vi "Actor Core.vi"(8 "error in":errorcluster, 11 "State in":refnum<class "System Actor.lvclass">) -> (0 "error out":errorcluster, 3 "Actor out":refnum<class "Actor.lvclass">)   [LabVIEW 2013, in "Robot Actors.lvlib" / "System Actor.lvlib" / "System Actor.lvclass"]
doc: "(<B>Filename</B>: Actor Framework.lvlib:Actor.lvclass:Actor Core.vi)\n\nThis override invokes Entry.vi on the initial state, prior to calling the parent Actor Core. Adding this behavior to Actor Core (instead of an override of Pre Launch Init.vi) allows the initial state to launch a nested actor as part of its entry behavior.\n\nReceives messages to the actor, reacts to them, and initiates any error handling that may shut the actor down.\n\nDescendant classes may override this VI to append parallel tasks for the actor to complete while it handles messages. Overrides use the Call Parent Method node."
uses:
  System Actor.lvclass
  State Actor/State Actor.lvclass
  <vilib>/ActorFramework/Actor/Actor.lvclass
  Command Processor/States/No Command/No Command Class/No Command.lvclass
  System Status.ctl
  Command/Command Class/Command Status.ctl
  Command/Command Class/Command.lvclass
  Command/Command Class/Command States.ctl
  Command Processor/Command Processor Class/Command Processor Status.ctl
  Command Processor/Command Processor Class/Command Processor.lvclass
  Command Processor/Command Processor Class/Command Processor States.ctl
panel:
  out "System Status":T1
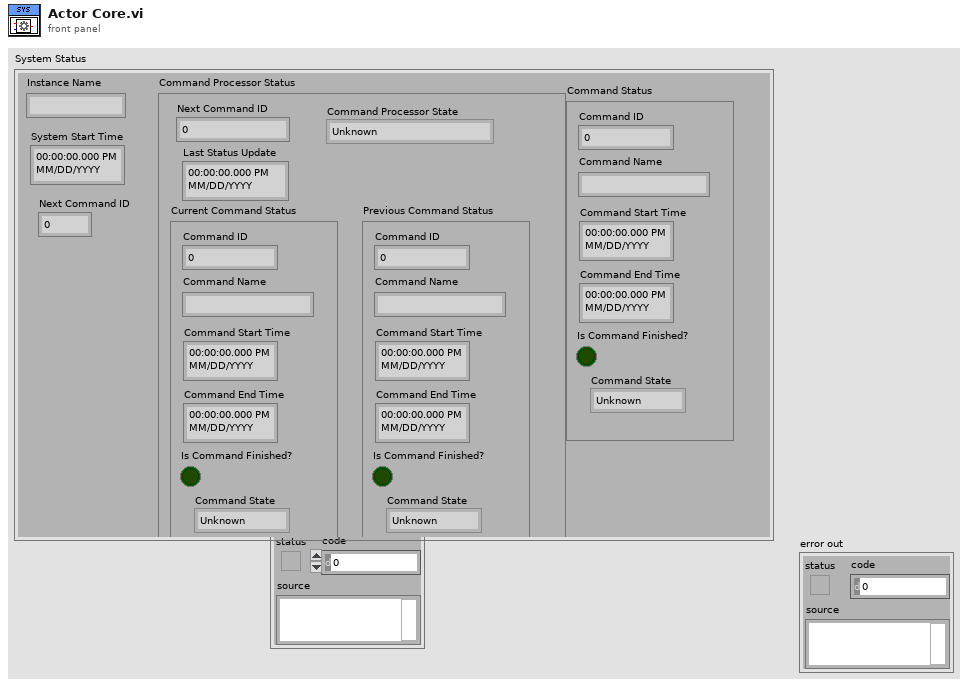
[diagram p1: front panel]
types:
  T1 = typedef "Robot Actors.lvlib/System Actor.lvlib/System Actor.lvclass/System Status.ctl" = cluster{"Instance Name":string, "Command Status":T2, "System Start Time":timestamp, "Next Command ID":dbl, "Command Processor Status":T4}
  T2 = typedef "Robot Actors.lvlib/Command.lvlib/Command.lvclass/Command Status.ctl" = cluster{"Command Name":string, "Command Start Time":timestamp, "Command End Time":timestamp, "Is Command Finished?":bool, "Command ID":dbl, "Command State":T3}
  T3 = typedef "Robot Actors.lvlib/Command.lvlib/Command.lvclass/Command States.ctl" = enum16{"Unknown", "Started", "Stopped", "Finished"}
  T4 = typedef "Robot Actors.lvlib/Command Processor.lvlib/Command Processor.lvclass/Command Processor Status.ctl" = cluster{"Next Command ID":dbl, "Current Command Status":T2, "Previous Command Status ":T2, "Command Processor State":T5, "Last Status Update":timestamp}
  T5 = typedef "Robot Actors.lvlib/Command Processor.lvlib/Command Processor.lvclass/Command Processor States.ctl" = enum16{"Unknown", "No Command", "Running Command"}
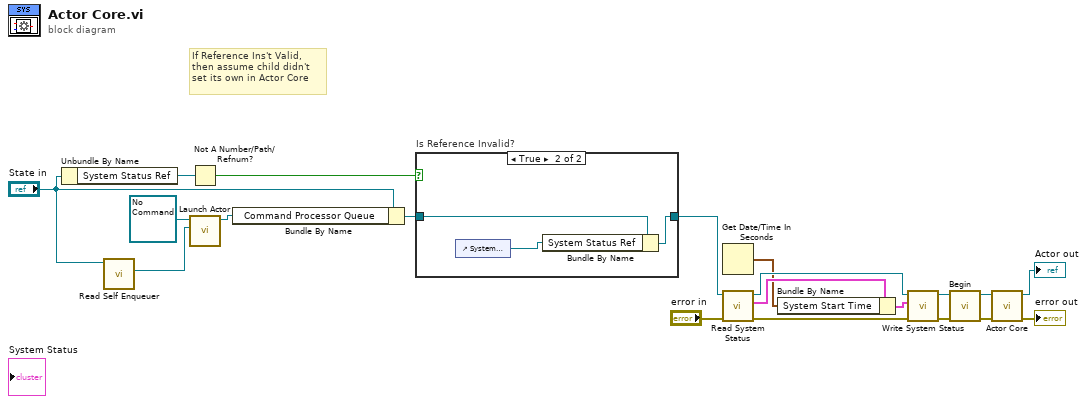
[diagram p0: block diagram]
diagram:
  # "If Reference Ins't Valid,\nthen assume child didn't \nset its own in Actor Core"
  n1 = Unbundle By Name("State in") -> ("System Status Ref"=w17:refnum<vi>)
  n2 = call <vilib>:"Read Self Enqueuer.vi"("Actor"="State in") -> ("Self Enqueuer"=w4:refnum<class "Message Enqueuer.lvclass">)  [unwired: 10 in]
  n3 = Not A Number/Path/Refnum?(number/path/refnum=w17) -> (NaN/Path/Refnum?=w16:bool)
  n4 = call <vilib>:"Launch Actor.vi"("Actor-to-Caller Enqueuer"=w4, "Actor"=refnum<class "No Command.lvclass"> refnum ("Robot Actors.lvlib:Command Processor.lvlib:No Command.lvclass")) -> ("Caller-To-Actor Enqueuer"=w2:refnum<class "Message Enqueuer.lvclass">)  [unwired: 8 in, 1 out]
  n5 = Bundle By Name(cluster="State in", "Command Processor Queue"=w2) -> (w3:refnum<class "System Actor.lvclass">)
  n6 = case "Is Reference Invalid?" shown="True" w16 {
    tunnel: w3 -> [w21 w24]
    tunnel: [w21 w23] -> w15
    frame False {
    }
    frame True {
      n7 = control-ref of="System Status"() -> (w22:refnum<vi>)
      n8 = Bundle By Name(cluster=w24, "System Status Ref"=w22) -> (w23:refnum<class "System Actor.lvclass">)
    }
  }
  n9 = Get Date/Time In Seconds() -> (seconds since 1Jan1904=w10:timestamp)
  n10 = call-dynamic "Read System Status.vi"("error in (no error)"="error in", "System Actor in"=w15) -> ("error out"=w8:errorcluster, "System Status"=w12:T1, "System Actor out"=w14:refnum<class "System Actor.lvclass">)  [unwired: 7 in]
  n11 = Bundle By Name(cluster=w12, "System Start Time"=w10) -> (w11:T1)
  n12 = call-dynamic "Write System Status.vi"("error in (no error)"=w8, "System Status"=w11, "System Actor in"=w14) -> ("error out"=w7:errorcluster, "System Actor out"=w13:refnum<class "System Actor.lvclass">)  [unwired: 7 in]
  n13 = call-dynamic "Begin.vi"("error in (no error)"=w7, "System Actor in"=w13) -> ("error out"=w6:errorcluster, "System Actor out"=w18:refnum<class "System Actor.lvclass">)  [unwired: 8 in]
  n14 = call-parent "Actor Core.vi"("error in"=w6, "State in"=w18) -> ("error out"=→"error out":errorcluster, "Actor out"=→"Actor out":refnum<class "Actor.lvclass">)  [unwired: 8 in]
